vi "check_run_settings.vi"(1 "Last Run Settings":T1={"Operator"="", "Sample (or CRM) ID"="", "Sample Temp"=0.0, "Salinity"=0.0, "Sample Units"=FALSE, "Sample Size"=0.0, "Operation Mode"=TRUE}, 2 "Current Run Settings":T1={"Operator"="", "Sample (or CRM) ID"="", "Sample Temp"=0.0, "Salinity"=0.0, "Sample Units"=FALSE, "Sample Size"=0.0, "Operation Mode"=TRUE}) -> (0 "New Run Settings":T1={"Operator"="", "Sample (or CRM) ID"="", "Sample Temp"=0.0, "Salinity"=0.0, "Sample Units"=FALSE, "Sample Size"=0.0, "Operation Mode"=TRUE})   [LabVIEW 2010]
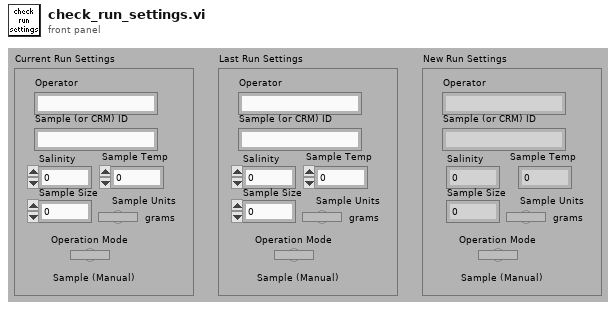
[diagram p1: front panel]
types:
  T1 = cluster{"Operator":string, "Sample (or CRM) ID":string, "Sample Temp":dbl, "Salinity":dbl, "Sample Units":bool, "Sample Size":dbl, "Operation Mode":bool}
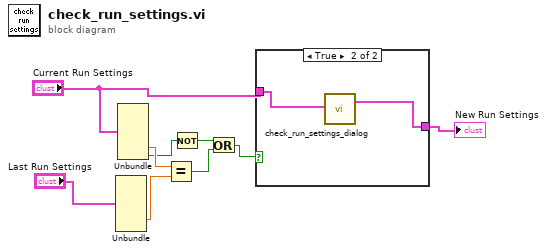
[diagram p0: block diagram]
diagram:
  n1 = Unbundle("Last Run Settings") -> ("Sample Size"=w5:dbl)  [unwired: 6 out]
  n2 = Unbundle("Current Run Settings") -> ("Sample Size"=w6:dbl, "Operation Mode"=w4:bool)  [unwired: 5 out]
  n3 = Equal?(x=w6, y=w5) -> (x = y?=w3:bool)
  n4 = Not(x=w4) -> (.not. x?=w2:bool)
  n5 = Or(x=w2, y=w3) -> (x .or. y?=w1:bool)
  n6 = case shown="True" w1 {
    tunnel: [w10 w11] -> w9
    tunnel: "Current Run Settings" -> [w10 w12]
    frame False {
    }
    frame True {
      n7 = call "check_run_settings_dialog.vi"("Current Run Settings"=w12) -> ("New Run Settings"=w11:T1)  [unwired: 16 in, 2 out]
    }
  }
  "New Run Settings" <- w9
